vi "Eurotherm - VISA Serial - Command.vi"(0 "VISA resource name In (String)":T1={"Com Port"=1, "Address"=1, "Baud Rate"=9600} {"Baud Rate" items=["300"=300, "600"=600, "1200"=1200, "2400"=2400, "4800"=4800, "9600 (default)"=9600, "19200"=19200, "38400"=38400, "57600"=57600, "76800"=76800, "115200"=115200, "230400"=230400]; "Com Port" min=1 max=255; "Address" min=1 max=99}, 5 "Command":string, 7 "Read Reply":bool, 9 "Close Session":bool, 11 "error in (no error)":errorcluster) -> (4 "VISA resource name Out (String)":T1={"Com Port"=1, "Address"=1, "Baud Rate"=9600} {"Baud Rate" items=["300"=300, "600"=600, "1200"=1200, "2400"=2400, "4800"=4800, "9600 (default)"=9600, "19200"=19200, "38400"=38400, "57600"=57600, "76800"=76800, "115200"=115200, "230400"=230400]; "Com Port" min=1 max=255; "Address" min=1 max=99}, 6 "Reply":string, 15 "error out":errorcluster)   [LabVIEW 2011]
uses:
  Eurotherm - Controls/Eurotherm - Communication.ctl
  Common/Utilities/Controls - Com Ports/Com Port - Numeric.ctl
  Eurotherm - Controls/Eurotherm - Address.ctl
  Common/Utilities/Controls - Com Ports/Com Port - Baud Rate.ctl
  Common/Utilities/Error Log/Error Log - Priority.ctl
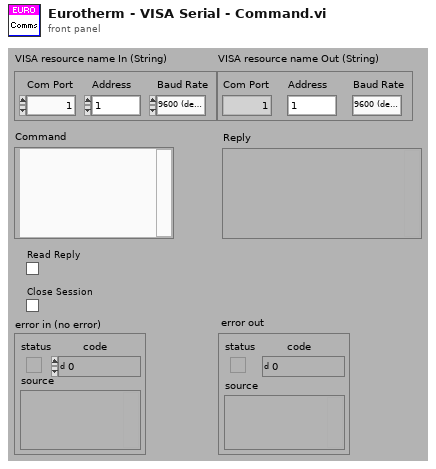
[diagram p1: front panel]
types:
  T1 = typedef "Eurotherm - Communication.ctl" = cluster{"Com Port":T2, "Address":T3, "Baud Rate":T4}
  T2 = typedef "Com Port - Numeric.ctl" = i32
  T3 = typedef "Eurotherm - Address.ctl" = u8
  T4 = typedef "Com Port - Baud Rate.ctl" = u32
  T5 = typedef "Error Log - Priority.ctl" = enum16{"None", "Log", "SECI and Log"}
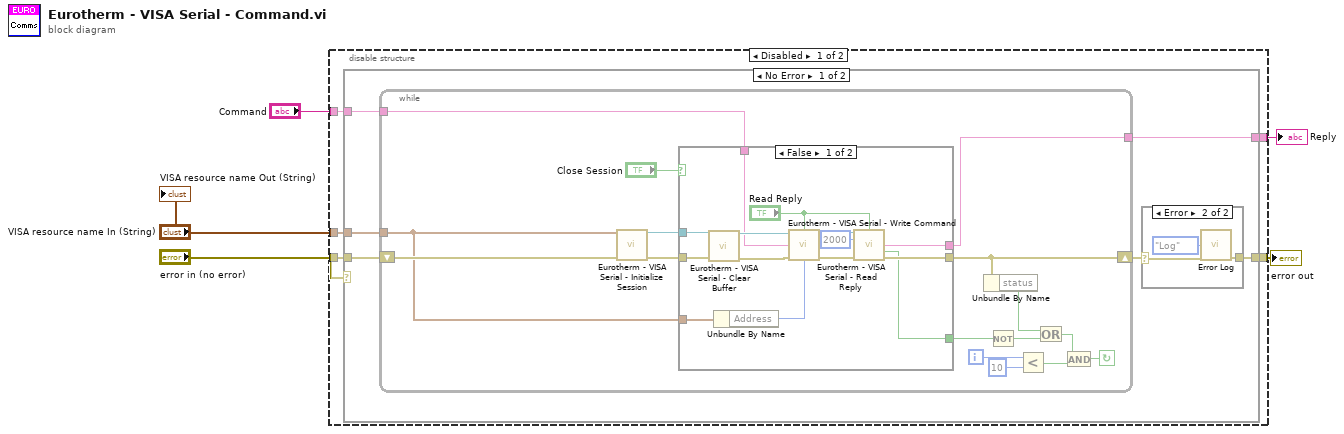
[diagram p0: block diagram]
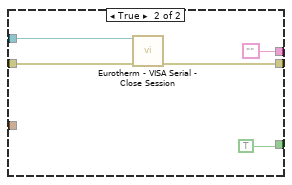
[diagram p3: hidden frame]
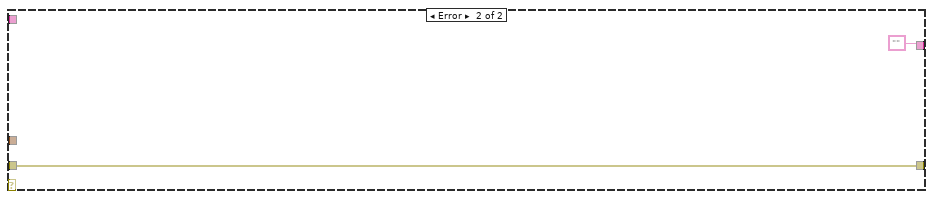
[diagram p4: hidden frame]
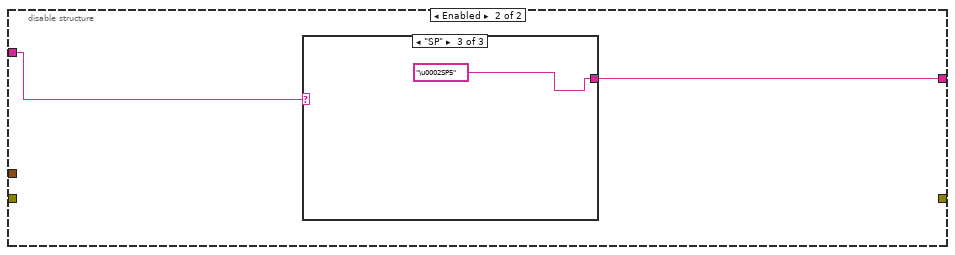
[diagram p5: hidden frame]
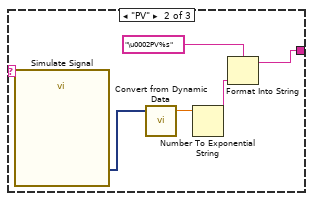
[diagram p7: hidden frame]
diagram:
  n1 = disable-structure shown="Disabled" {
    disable-tunnel: "VISA resource name In (String)" -> [w10 _]
    disable-tunnel: [w9 _] -> w4
    disable-tunnel: "error in (no error)" -> [w8 _]
    disable-tunnel: [w7 w58] -> w2
    disable-tunnel: "Command" -> [w6 w59]
    frame Disabled {
      n2 = case shown="No Error" w8 {
        tunnel: w8 -> [w16 w57]
        tunnel: w10 -> [w15 _]
        tunnel: [w13 w57] -> w9
        tunnel: [w12 ""] -> w7
        tunnel: w6 -> [w11 _]
        frame No Error {
          n3 = while {
            shift-right: [w30] -> w14
            shift-left: w16 -> [w34]
            tunnel: w15 -> [w23]
            tunnel: [w22] -> w12
            tunnel: w11 -> [w21]
            i -> [w36]
            stop <- w29 continue-if-true
            n4 = call "Eurotherm - VISA Serial - Initialize Session.vi"("Communication"=w23, "error in (no error)"=w34) -> ("VISA"=w32:refnum<visa-resource-name>, "error out"=w33:errorcluster)  [unwired: 12 in]
            n5 = case shown="False" "Close Session" {
              tunnel: w33 -> [w44 w54]
              tunnel: w32 -> [w45 w53]
              tunnel: [w47 w55] -> w30
              tunnel: [w48 ""] -> w22
              tunnel: [w46 TRUE] -> w25
              tunnel: w23 -> [w40 _]
              tunnel: w21 -> [w37 _]
              frame False {
                n6 = call "Eurotherm - VISA Serial - Clear Buffer.vi"("VISA resource name"=w45, "error in (no error)"=w44) -> ("dup VISA resource name"=w42:refnum<visa-resource-name>, "error out"=w43:errorcluster)  [unwired: 12 in]
                n7 = Unbundle By Name(w40) -> ("Address"=w39:T3)
                n8 = call "Eurotherm - VISA Serial - Write Command.vi"("VISA resource name"=w42, "Read Reply"="Read Reply", "write buffer"=w37, "error in (no error)"=w43, "Address"=w39) -> ("dup VISA resource name"=w49:refnum<visa-resource-name>, "error out"=w50:errorcluster)  [unwired: 8 in, 1 out]
                n9 = call "Eurotherm - VISA Serial - Read Reply.vi"("VISA resource name"=w49, "Read Reply"="Read Reply", "Timeout (ms)"=u32 2000, "error in (no error)"=w50) -> ("read buffer"=w48:string, "Success"=w46:bool, "error out"=w47:errorcluster)  [unwired: 8 in, 1 out]
              }
              frame True {
                n10 = call "Eurotherm - VISA Serial - Close Session.vi"("VISA resource name"=w53, "error in (no error)"=w54) -> ("error out"=w55:errorcluster)  [unwired: 12 in, 1 out]
              }
            }
            n11 = Unbundle By Name(w30) -> ("status"=w26:bool)
            n12 = Not(x=w25) -> (.not. x?=w24:bool)
            n13 = Less?(x=w36, y=10) -> (x < y?=w28:bool)
            n14 = Or(x=w26, y=w24) -> (x .or. y?=w27:bool)
            n15 = And(x=w27, y=w28) -> (x .and. y?=w29:bool)
          }
          n16 = case shown="Error" w14 {
            selector: w14 -> [w17 w19]
            tunnel: [w17 w18] -> w13
            frame No Error {
            }
            frame Error {
              n17 = call "Error Log.vi"("Priority"=Error_Log_-_Priority."Log", "error in (no error)"=w19) -> ("error out"=w18:errorcluster)  [unwired: 13 in]
            }
          }
        }
        frame Error {
        }
      }
    }
    frame Enabled {
      n18 = case shown="\"SP\"" w59 {
        selector: w59 -> [w60 _ _]
        tunnel: [w60 w64 "\u0002SP5"] -> w58
        frame Default {
        }
        frame "PV" {
          n19 = call "Simulate Signal"() -> ("Sine with Uniform Noise"=w62:dynamicdata)  [unwired: 14 in, 1 out]
          n20 = call "Convert from Dynamic Data"("Dynamic Data Type"=w62) -> ("Scalar"=w63:dbl)  [unwired: 3 in]
          n21 = Number To Exponential String(number=w63) -> (E-format string=w61:string)  [unwired: 3 in]
          n22 = Format Into String(format string="\u0002PV%s", w61) -> (resulting string=w64:string)  [unwired: 2 in, 1 out]
        }
        frame "SP" {
        }
      }
    }
  }
  "error out" <- w4
  "Reply" <- w2
  "VISA resource name Out (String)" <- "VISA resource name In (String)"
